vi "CRYGet Channel Array.vi"(11 "Channel Array":T1[](array[typedef]) {"Coupling" items=["Default"=-1, "RSE"=10083, "NRSE"=10078, "Differential"=10106, "Pseudodifferential"=12529]; "term config" items=["Default"=-1, "RSE"=10083, "NRSE"=10078, "Differential"=10106, "Pseudodifferential"=12529]; "Anti-aliasing Factor (%fs)" format="%.2f"}) -> (0 "I Channel Info Out":T1[](array[typedef]) {"Coupling" items=["Default"=-1, "RSE"=10083, "NRSE"=10078, "Differential"=10106, "Pseudodifferential"=12529]; "term config" items=["Default"=-1, "RSE"=10083, "NRSE"=10078, "Differential"=10106, "Pseudodifferential"=12529]; "Anti-aliasing Factor (%fs)" format="%.2f"}, 1 "I_Channel Name Out":string[](array[string]), 2 "O Channel Info Out":T1[](array[typedef]) {"Coupling" items=["Default"=-1, "RSE"=10083, "NRSE"=10078, "Differential"=10106, "Pseudodifferential"=12529]; "term config" items=["Default"=-1, "RSE"=10083, "NRSE"=10078, "Differential"=10106, "Pseudodifferential"=12529]; "Anti-aliasing Factor (%fs)" format="%.2f"}, 3 "O_Channel Name Out":string[](array[string]))   [LabVIEW 2013]
uses:
  Typedef Control/CRYHardware Channel Info.ctl
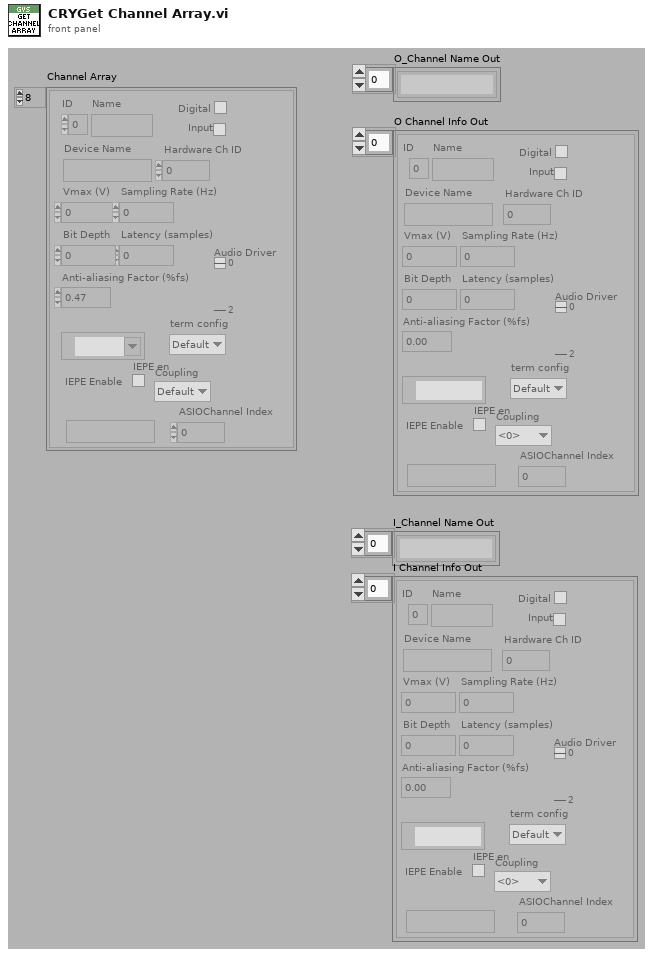
[diagram p1: front panel]
types:
  T1 = typedef "CRYHardware Channel Info.ctl" = cluster{"ID":i32, "Name":string, "Digital":bool, "Input":bool, "Device Name":string, "Hardware Ch ID":u8, "Vmax (V)":dbl, "Latency (samples)":dbl, "Sampling Rate (Hz)":u32, "Bit Depth":u32, "Anti-aliasing Factor (%fs)":sgl, "DAQmx Channel":tag, "term config":i32, "Coupling":i32, "IEPE en":bool, "ASIOChannel Name":string, "Audio Driver":u16, "ASIOChannel Index":u8}
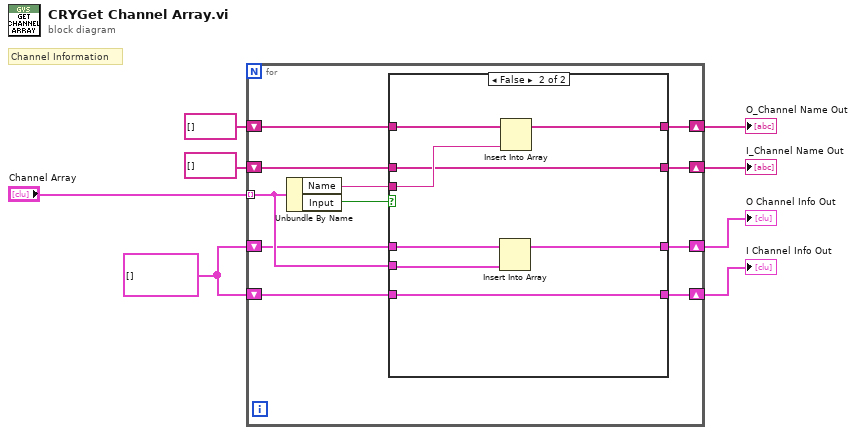
[diagram p0: block diagram]
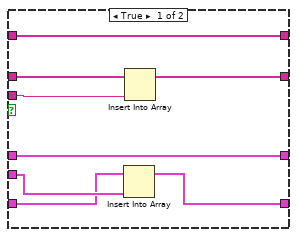
[diagram p2: hidden frame]
diagram:
  w6 = T1[] []
  # "Channel Information"
  n1 = for {
    tunnel: "Channel Array" -> [w13] mode=indexing
    shift-right: [w18] -> w5
    shift-left: string[] [] -> [w17]
    shift-right: [w14] -> w4
    shift-left: string[] [] -> [w15]
    shift-right: [w12] -> w3
    shift-left: w6 -> [w11]
    shift-right: [w10] -> w2
    shift-left: w6 -> [w9]
    n2 = Unbundle By Name(w13) -> ("Name"=w19:string, "Input"=w16:bool)
    n3 = case shown="False" w16 {
      tunnel: w19 -> [w27 w35]
      tunnel: [w24 w34] -> w18
      tunnel: w17 -> [w24 w33]
      tunnel: w15 -> [w26 w32]
      tunnel: [w25 w32] -> w14
      tunnel: w13 -> [w22 w31]
      tunnel: [w23 w30] -> w12
      tunnel: w11 -> [w23 w29]
      tunnel: [w21 w28] -> w10
      tunnel: w9 -> [w20 w28]
      frame True {
        n4 = Insert Into Array(array=w20, new element=w22) -> (w21:T1[])  [unwired: 1 in]
        n5 = Insert Into Array(array=w26, new element=w27) -> (w25:string[])  [unwired: 1 in]
      }
      frame False {
        n6 = Insert Into Array(array=w29, new element=w31) -> (w30:T1[])  [unwired: 1 in]
        n7 = Insert Into Array(array=w33, new element=w35) -> (w34:string[])  [unwired: 1 in]
      }
    }
  }
  "O_Channel Name Out" <- w5
  "I_Channel Name Out" <- w4
  "O Channel Info Out" <- w3
  "I Channel Info Out" <- w2
